vi "Set Motor Toque.vi"(6 "error in":errorcluster, 7 "FloatNumber":sgl, 8 "MaxRead":i32, 9 "Channel in":u16) -> (0 "error out":errorcluster, 1 "Messages":T1(array[cluster]) {"DATA[0]" format="%.0x"; "DATA[1]" format="%.0x"; "DATA[2]" format="%.0x"; "DATA[3]" format="%.0x"; "DATA[4]" format="%.0x"; "DATA[5]" format="%.0x"; "DATA[6]" format="%.0x"; "DATA[7]" format="%.0x"}, 2 "Pass":bool, 3 "Channel out":u16)   [LabVIEW 2023]
uses:
  df35a301-8fcb-495c-91e3-c82146f18b8b.vi
  57138545-9434-49a5-ae43-5830d40555d7.vi
  14c262b7-9e9c-492d-9131-308f2605586c.vi
  77ee3bd8-ee1b-40a1-81ef-9bf9d5483e65.vi
  2ad30504-fef7-4a6b-a16d-0a474ce5601d.vi
  e99ada8f-d09f-4018-ada1-fc308b247a31.vi
  Communication/PCAN2023/PCAN API.lvlib
panel:
  out "Messages 2":T1(array[cluster]) {"DATA[0]" format="%.0x"; "DATA[1]" format="%.0x"; "DATA[2]" format="%.0x"; "DATA[3]" format="%.0x"; "DATA[4]" format="%.0x"; "DATA[5]" format="%.0x"; "DATA[6]" format="%.0x"; "DATA[7]" format="%.0x"}
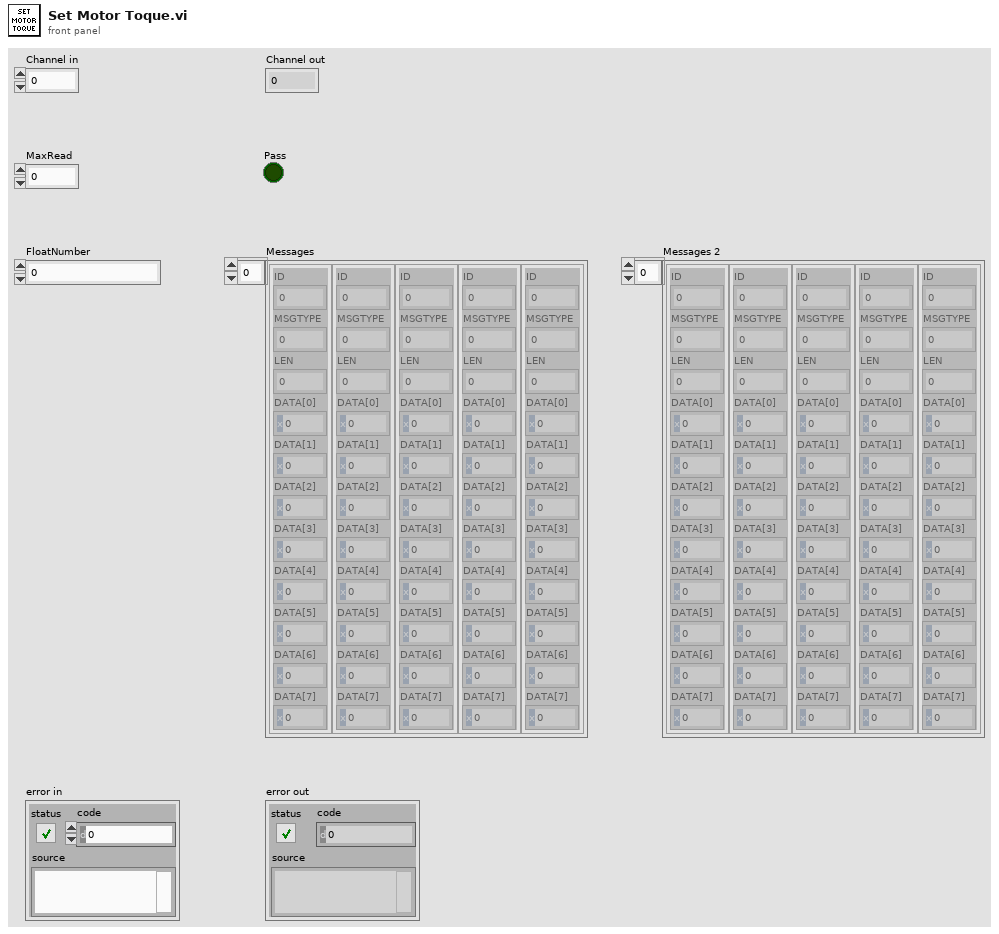
[diagram p1: front panel]
types:
  T1 = cluster{"ID":u32, "MSGTYPE":u8, "LEN":u8, "DATA[0]":u8, "DATA[1]":u8, "DATA[2]":u8, "DATA[3]":u8, "DATA[4]":u8, "DATA[5]":u8, "DATA[6]":u8, "DATA[7]":u8}[]
  T2 = cluster{"ID":u32, "MSGTYPE":u8, "LEN":u8, "DATA[0]":u8, "DATA[1]":u8, "DATA[2]":u8, "DATA[3]":u8, "DATA[4]":u8, "DATA[5]":u8, "DATA[6]":u8, "DATA[7]":u8}
  T3 = cluster{"ID":bool, "MSGTYPE":bool, "LEN":bool, "DATA[0]":bool, "DATA[1]":bool, "DATA[2]":bool, "DATA[3]":bool, "DATA[4]":bool, "DATA[5]":bool, "DATA[6]":bool, "DATA[7]":bool}
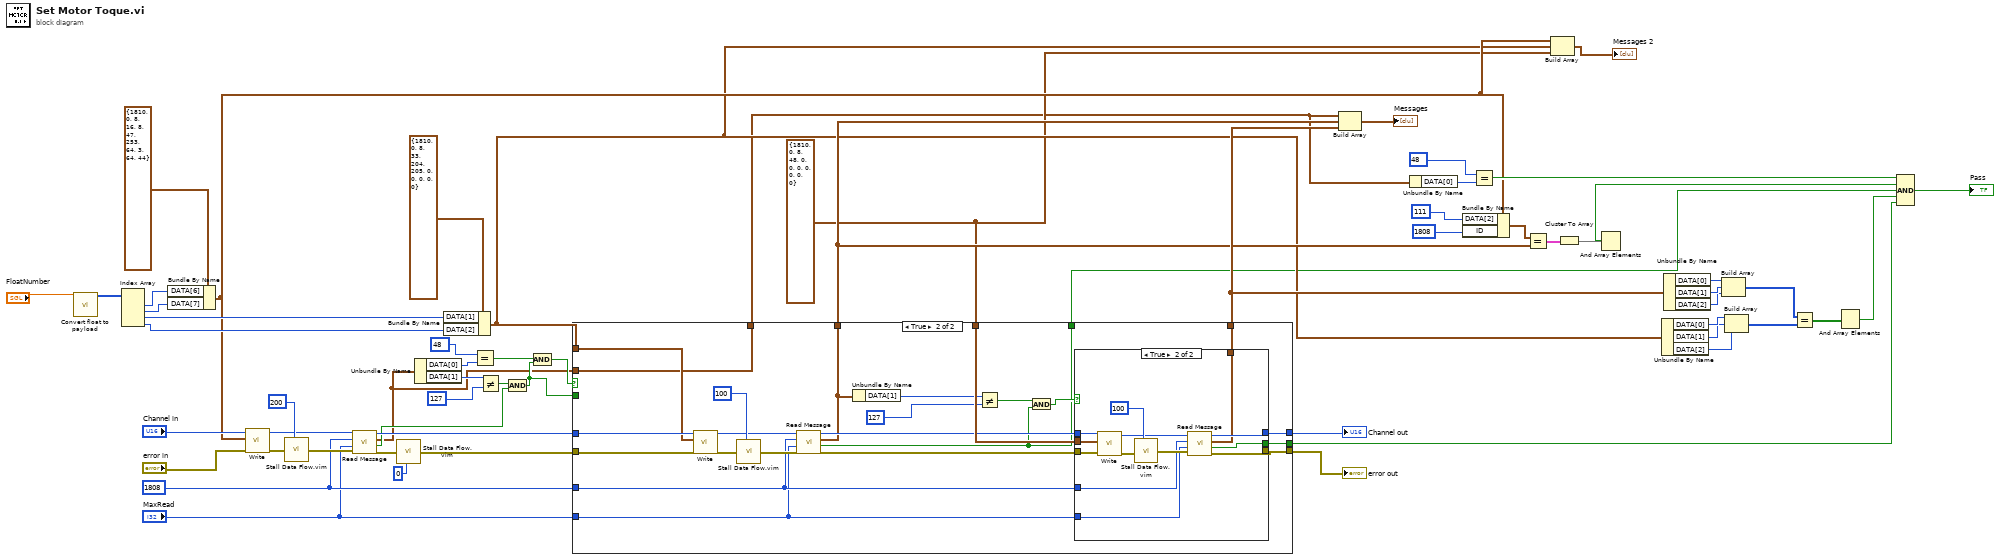
[diagram p0: block diagram]
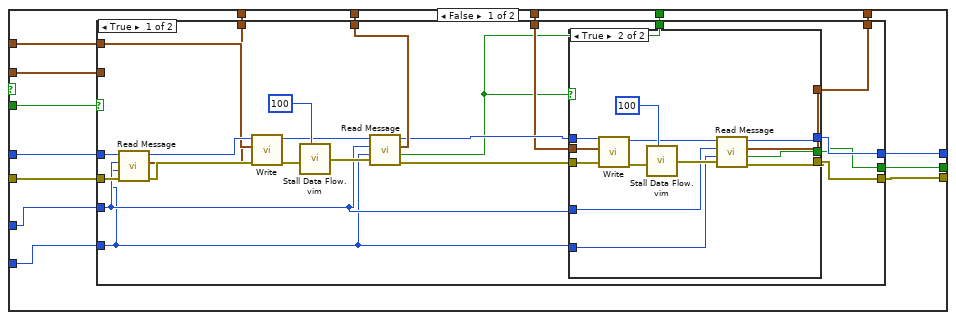
[diagram p2: hidden frame]
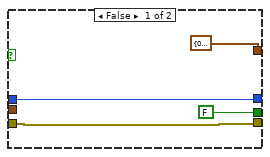
[diagram p3: hidden frame]
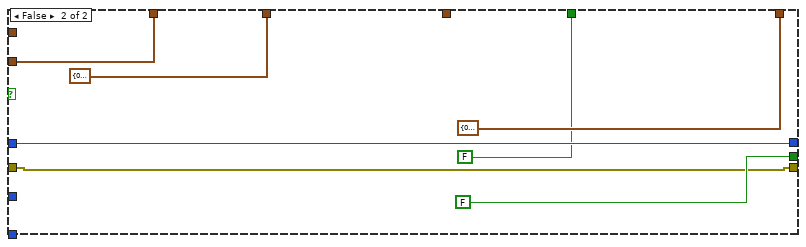
[diagram p4: hidden frame]
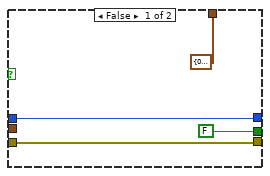
[diagram p5: hidden frame]
diagram:
  w11 = T2 {"ID"=1810, "MSGTYPE"=0, "LEN"=8, "DATA[0]"=48, "DATA[1]"=0, "DATA[2]"=0, "DATA[3]"=0, "DATA[4]"=0, "DATA[5]"=0, "DATA[6]"=0, "DATA[7]"=0} ("MessageBuffer")
  w16 = u32 1808 ("ID")
  n1 = call "Convert float to payload.vi"("FloatNumber"="FloatNumber") -> ("Converted Payload"=w52:u8[])  [unwired: 18 in]
  n2 = Index Array(array=w52) -> (element #1=w51:u8, element #2=w50:u8, element #3=w48:u8, element #4=w47:u8)  [unwired: 4 in]
  n3 = Bundle By Name(cluster=T2 {"ID"=1810, "MSGTYPE"=0, "LEN"=8, "DATA[0]"=16, "DATA[1]"=8, "DATA[2]"=47, "DATA[3]"=253, "DATA[4]"=64, "DATA[5]"=3, "DATA[6]"=64, "DATA[7]"=44} ("MessageBuffer"), "DATA[6]"=w51, "DATA[7]"=w50) -> (w13:T2)
  n4 = call "Write.vi"("error in"="error in", "MessageBuffer"=w13, "Channel"="Channel in") -> ("error out"=w61:errorcluster, "Channel out"=w20:u16)  [unwired: 5 in, 2 out]
  n5 = call "Stall Data Flow.vim"("value in"=w61, "milliseconds to wait"=u32 200) -> ("value out"=w19:errorcluster)  [unwired: 1 out]
  n6 = call "Read Message.vi"("error in"=w19, "MaxRead"="MaxRead", "ID"=w16, "Channel in"=w20) -> ("error out"=w17:errorcluster, "Passed"=w10:bool, "Last Message"=w3:T2, "Channel out"=w18:u16)  [unwired: 3 in, 1 out]
  n7 = call "Stall Data Flow.vim"("value in"=w17, "milliseconds to wait"=u32 0) -> ("value out"=w59:errorcluster)  [unwired: 1 out]
  n8 = Unbundle By Name(w3) -> ("DATA[0]"=w9:u8, "DATA[1]"=w23:u8)
  n9 = Bundle By Name(cluster=T2 {"ID"=1810, "MSGTYPE"=0, "LEN"=8, "DATA[0]"=33, "DATA[1]"=204, "DATA[2]"=205, "DATA[3]"=0, "DATA[4]"=0, "DATA[5]"=0, "DATA[6]"=0, "DATA[7]"=0} ("MessageBuffer"), "DATA[1]"=w48, "DATA[2]"=w47) -> (w12:T2)
  n10 = Equal?(x=u8 48 ("y"), y=w9) -> (x = y?=w6:bool)
  n11 = Not Equal?(x=w23, y=u8 127) -> (x != y?=w7:bool)
  n12 = And(x=w7, y=w10) -> (x .and. y?=w4:bool)
  n13 = And(x=w6, y=w4) -> (x .and. y?=w5:bool)
  n14 = case shown="True" w5 {
    tunnel: w18 -> [w72 w144]
    tunnel: w59 -> [w71 w143]
    tunnel: w11 -> [w67 w141]
    tunnel: w12 -> [w70 w140]
    tunnel: [w64 w139] -> w21
    tunnel: [w66 w138] -> w35
    tunnel: [w65 w137] -> w34
    tunnel: [w76 w136] -> w29
    tunnel: [w77 w129] -> w22
    tunnel: w16 -> [w69 w128]
    tunnel: "MaxRead" -> [w68 w127]
    tunnel: w4 -> [w75 _]
    tunnel: w3 -> [w74 w124]
    tunnel: [w73 w124] -> w2
    tunnel: [w63 w123] -> w1
    frame False {
      n15 = case shown="True" w75 {
        tunnel: [w88 T2 {"ID"=0, "MSGTYPE"=0, "LEN"=0, "DATA[0]"=0, "DATA[1]"=0, "DATA[2]"=0, "DATA[3]"=0, "DATA[4]"=0, "DATA[5]"=0, "DATA[6]"=0, "DATA[7]"=0} ("MessageBuffer out")] -> w77
        tunnel: [w84 T2 {"ID"=0, "MSGTYPE"=0, "LEN"=0, "DATA[0]"=0, "DATA[1]"=0, "DATA[2]"=0, "DATA[3]"=0, "DATA[4]"=0, "DATA[5]"=0, "DATA[6]"=0, "DATA[7]"=0} ("MessageBuffer out")] -> w76
        tunnel: [w81 FALSE] -> w64
        tunnel: w74 -> [_ w119]
        tunnel: [w89 w119] -> w73
        tunnel: w72 -> [w98 w118]
        tunnel: w71 -> [w97 w117]
        tunnel: w70 -> [w90 _]
        tunnel: w69 -> [w79 _]
        tunnel: w68 -> [w78 _]
        tunnel: w67 -> [w86 _]
        tunnel: [w83 w118] -> w65
        tunnel: [w82 w117] -> w66
        tunnel: [w80 FALSE] -> w63
        frame True {
          n16 = call "Read Message.vi"("error in"=w97, "MaxRead"=w78, "ID"=w79, "Channel in"=w98) -> ("error out"=w91:errorcluster, "Last Message"=w89:T2, "Channel out"=w92:u16)  [unwired: 3 in, 2 out]
          n17 = call "Write.vi"("error in"=w91, "MessageBuffer"=w90, "Channel"=w92) -> ("error out"=w96:errorcluster, "Channel out"=w94:u16)  [unwired: 5 in, 2 out]
          n18 = call "Stall Data Flow.vim"("value in"=w96, "milliseconds to wait"=u32 100) -> ("value out"=w93:errorcluster)  [unwired: 1 out]
          n19 = call "Read Message.vi"("error in"=w93, "MaxRead"=w78, "ID"=w79, "Channel in"=w94) -> ("error out"=w85:errorcluster, "Passed"=w80:bool, "Last Message"=w88:T2, "Channel out"=w87:u16)  [unwired: 3 in, 1 out]
          n20 = case shown="True" w80 {
            tunnel: w87 -> [w102 w115]
            tunnel: w86 -> [_ w114]
            tunnel: [FALSE w107] -> w81
            tunnel: [w99 w108] -> w82
            tunnel: [w102 w109] -> w83
            tunnel: [T2 {"ID"=0, "MSGTYPE"=0, "LEN"=0, "DATA[0]"=0, "DATA[1]"=0, "DATA[2]"=0, "DATA[3]"=0, "DATA[4]"=0, "DATA[5]"=0, "DATA[6]"=0, "DATA[7]"=0} ("MessageBuffer out") w106] -> w84
            tunnel: w79 -> [_ w105]
            tunnel: w78 -> [_ w104]
            tunnel: w85 -> [w99 w103]
            frame False {
            }
            frame True {
              n21 = call "Write.vi"("error in"=w103, "MessageBuffer"=w114, "Channel"=w115) -> ("error out"=w113:errorcluster, "Channel out"=w111:u16)  [unwired: 5 in, 2 out]
              n22 = call "Stall Data Flow.vim"("value in"=w113, "milliseconds to wait"=u32 100) -> ("value out"=w110:errorcluster)  [unwired: 1 out]
              n23 = call "Read Message.vi"("error in"=w110, "MaxRead"=w104, "ID"=w105, "Channel in"=w111) -> ("error out"=w108:errorcluster, "Passed"=w107:bool, "Last Message"=w106:T2, "Channel out"=w109:u16)  [unwired: 3 in, 1 out]
            }
          }
        }
        frame False {
        }
      }
    }
    frame True {
      n24 = call "Write.vi"("error in"=w143, "MessageBuffer"=w140, "Channel"=w144) -> ("error out"=w145:errorcluster, "Channel out"=w133:u16)  [unwired: 5 in, 2 out]
      n25 = call "Stall Data Flow.vim"("value in"=w145, "milliseconds to wait"=u32 100) -> ("value out"=w132:errorcluster)  [unwired: 1 out]
      n26 = call "Read Message.vi"("error in"=w132, "MaxRead"=w127, "ID"=w128, "Channel in"=w133) -> ("error out"=w130:errorcluster, "Passed"=w123:bool, "Last Message"=w129:T2, "Channel out"=w131:u16)  [unwired: 3 in, 1 out]
      n27 = Unbundle By Name(w129) -> ("DATA[1]"=w134:u8)
      n28 = Not Equal?(x=w134, y=u8 127) -> (x != y?=w126:bool)
      n29 = And(x=w126, y=w123) -> (x .and. y?=w125:bool)
      n30 = case shown="True" w125 {
        tunnel: w131 -> [w149 w162]
        tunnel: w130 -> [w147 w161]
        tunnel: w141 -> [_ w160]
        tunnel: [FALSE w153] -> w139
        tunnel: [w147 w154] -> w138
        tunnel: [w149 w155] -> w137
        tunnel: [T2 {"ID"=0, "MSGTYPE"=0, "LEN"=0, "DATA[0]"=0, "DATA[1]"=0, "DATA[2]"=0, "DATA[3]"=0, "DATA[4]"=0, "DATA[5]"=0, "DATA[6]"=0, "DATA[7]"=0} ("MessageBuffer out") w152] -> w136
        tunnel: w128 -> [_ w151]
        tunnel: w127 -> [_ w150]
        frame False {
        }
        frame True {
          n31 = call "Write.vi"("error in"=w161, "MessageBuffer"=w160, "Channel"=w162) -> ("error out"=w159:errorcluster, "Channel out"=w157:u16)  [unwired: 5 in, 2 out]
          n32 = call "Stall Data Flow.vim"("value in"=w159, "milliseconds to wait"=u32 100) -> ("value out"=w156:errorcluster)  [unwired: 1 out]
          n33 = call "Read Message.vi"("error in"=w156, "MaxRead"=w150, "ID"=w151, "Channel in"=w157) -> ("error out"=w154:errorcluster, "Passed"=w153:bool, "Last Message"=w152:T2, "Channel out"=w155:u16)  [unwired: 3 in, 1 out]
        }
      }
    }
  }
  "error out" <- w35
  "Channel out" <- w34
  n34 = Build Array(w2, w22, w29) -> (→"Messages":T1)
  n35 = Unbundle By Name(w2) -> ("DATA[0]"=w46:u8)
  n36 = Bundle By Name(cluster=w13, "DATA[2]"=u8 111 ("x"), "ID"=u32 1808) -> (w28:T2)
  n37 = Equal?(x=u8 48, y=w46) -> (x = y?=w33:bool)
  n38 = Equal?(x=w28, y=w22) -> (x = y?=w32:T3)
  n39 = Build Array(w13, w12, w11) -> (→"Messages 2":T1)
  n40 = Cluster To Array(cluster=w32) -> (array=w31:bool[])
  n41 = And Array Elements(Boolean array=w31) -> (logical AND=w30:bool)
  n42 = Unbundle By Name(w12) -> ("DATA[0]"=w41:u8, "DATA[1]"=w40:u8, "DATA[2]"=w39:u8)
  n43 = Unbundle By Name(w29) -> ("DATA[0]"=w44:u8, "DATA[1]"=w43:u8, "DATA[2]"=w42:u8)
  n44 = Build Array(w44, w43, w42) -> (w38:u8[])
  n45 = Build Array(w41, w40, w39) -> (w37:u8[])
  n46 = Equal?(x=w38, y=w37) -> (x = y?=w36:bool[])
  n47 = And Array Elements(Boolean array=w36) -> (logical AND=w56:bool)
  n48 = Compound Arithmetic op=AND(w33, w30, w1, w56, w21) -> (→"Pass":bool)
